vi "RTS Build File Name Doors.vi"(8 "error in (no error)":errorcluster, 10 "File Name":string, 11 "Stripped Path Input":path) -> (0 "error out":errorcluster, 3 "appended path":path)   [LabVIEW 2016]
uses:
  <vilib>/Utility/config.llb/NI_LVConfig.lvlib
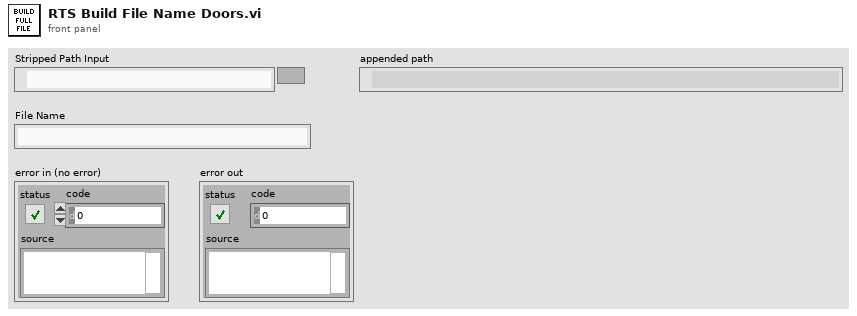
[diagram p1: front panel]
types:
  T1 = typedef "NI_LVConfig.lvlib/Config Data RefNum.ctl" = refnum<k1>
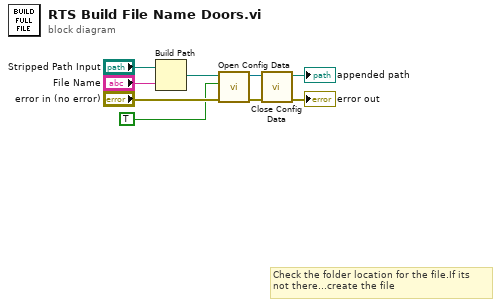
[diagram p0: block diagram]
diagram:
  # "Check the folder location for the file.If its \nnot there...create the file"
  n1 = Build Path(base path="Stripped Path Input", name or relative path="File Name") -> (appended path=w7:path)
  n2 = call <vilib>:"Open Config Data.vi"("error in (no error)"="error in (no error)", "create file if necessary (T)"=TRUE, "configuration file path"=w7) -> ("error out"=w2:errorcluster, "refnum"=w3:T1)  [unwired: 6 in, 1 out]
  n3 = call <vilib>:"Close Config Data.vi"("error in (no error)"=w2, "refnum"=w3) -> ("error out"=→"error out":errorcluster, "file path"=→"appended path":path)  [unwired: 8 in]
